vi "Extend Symbol Path_lvcicd.vi"(3 "Symbol Path":path) -> (1 "Resolved Path":path)   [LabVIEW 2014, in "_lvcicd_support_2014.lvlib"]
doc: "NEVSTOP-Programming-Palette 2022.3.9.1\nNEVSTOP - NEVSTOP\nCopyright (c) 2022, NEVSTOP"
uses:
  <vilib>/Utility/sysdir.llb/System Directory Type.ctl
  <userlib>/_OpenG.lib/file/file.llb/Valid Path - Traditional__ogtk.vi
  _lvcicd_support_2014.lvlib
  kernel32.dll
panel:
  # "#Note [xxx] or <xxx>\n- [application]\n- [desktop]\n- [temp][temporary]\n- [user.lib]\n- [vi.lib]\n-%SystemVariable%, eg: OneDrive"
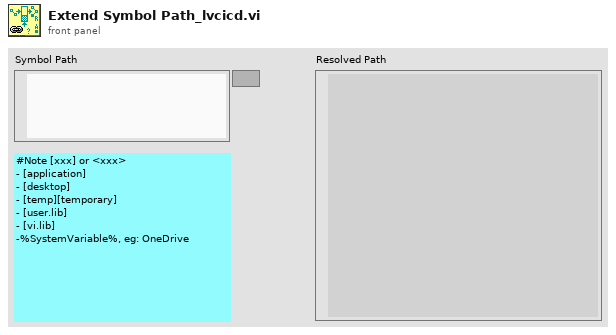
[diagram p1: front panel]
types:
  T1 = enum16{"Absolute path", "Relative path", "<Not A Path>"}
  T2 = typedef "System Directory Type.ctl" = i32
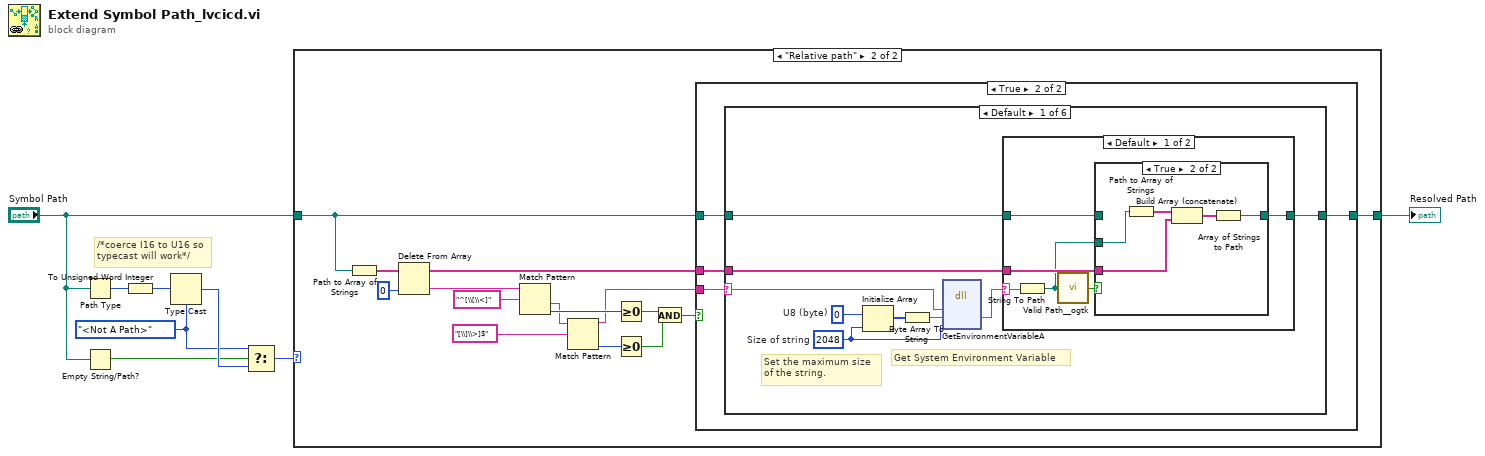
[diagram p0: block diagram]
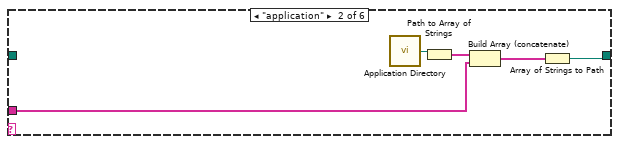
[diagram p6: hidden frame]
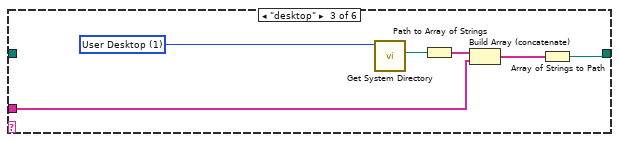
[diagram p7: hidden frame]
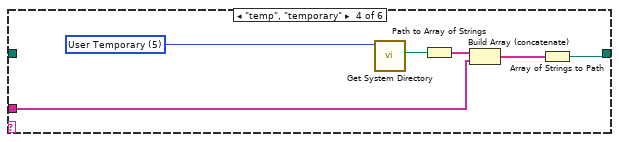
[diagram p8: hidden frame]
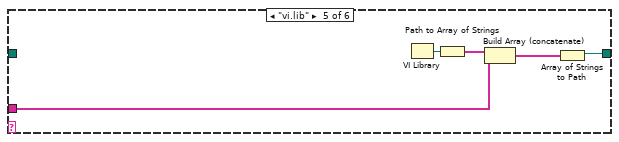
[diagram p9: hidden frame]
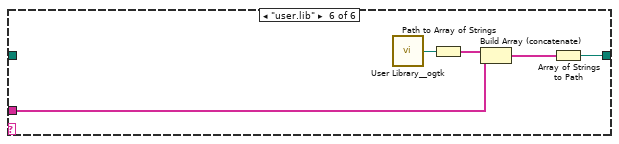
[diagram p10: hidden frame]
diagram:
  w3 = T1."<Not A Path>"
  # "/*coerce I16 to U16 so typecast will work*/"
  n1 = Path Type(1:"Symbol Path") -> (0:w1:i16)
  n2 = Empty String/Path?(string/path="Symbol Path") -> (empty?=w2:bool)
  n3 = To Unsigned Word Integer(number=w1) -> (unsigned 16bit integer=w5:u16)
  n4 = Type Cast(type=w3, x=w5) -> (*(type *) &x=w4:T1)
  n5 = Select(t=w3, s=w2, f=w4) -> (s? t:f=w8:T1)
  n6 = case shown="\"Relative path\"" w8 {
    tunnel: [w9 w16] -> w7
    tunnel: "Symbol Path" -> [w9 w15]
    frame "Absolute path", "<Not A Path>", Default {
    }
    frame "Relative path" {
      n7 = Path to Array of Strings(0:w15) -> (2:w24:string[])  [unwired: 1 out]
      n8 = Delete From Array(array=w24, index=0) -> (deleted portion=w14:string, array with subset deleted=w10:string[])  [unwired: 1 in]
      n9 = Match Pattern(string=w14, regular expression="^[\\[\\<]") -> (after substring=w13:string, offset past match=w21:i32)  [unwired: 1 in, 2 out]
      n10 = Match Pattern(string=w13, regular expression="[\\]\\>]$") -> (before substring=w12:string, offset past match=w20:i32)  [unwired: 1 in, 2 out]
      n11 = Greater Or Equal To 0?(x=w21) -> (x >= 0?=w19:bool)
      n12 = Greater Or Equal To 0?(x=w20) -> (x >= 0?=w18:bool)
      n13 = And(x=w19, y=w18) -> (x .and. y?=w17:bool)
      n14 = case shown="True" w17 {
        tunnel: [w25 w26] -> w16
        tunnel: w15 -> [w25 w28]
        tunnel: w12 -> [_ w29]
        tunnel: w10 -> [_ w27]
        frame False {
        }
        frame True {
          n15 = case shown="Default" w29 {
            selector: w29 -> [w38 _ _ _ _ _]
            tunnel: w28 -> [w35 _ _ _ _ _]
            tunnel: w27 -> [w34 w52 w59 w65 w69 w74]
            tunnel: [w36 w54 w60 w66 w71 w76] -> w26
            frame Default {
              w31 = u8 0  # U8 (byte)
              w30 = 2048  # Size of string
              # "Set the maximum size\nof the string."
              # "Get System Environment Variable"
              n16 = Initialize Array(w31, w30) -> (w32:u8[])
              n17 = Byte Array To String(unsigned byte array=w32) -> (string=w33:string)
              n18 = dll-call lib="kernel32.dll" fn="GetEnvironmentVariableA"("EnvVarName"=w38, "lpBuffer"=w33, "namelength"=w30) -> ("lpBuffer"=w37:string)  [unwired: 6 in, 2 out]
              n19 = case shown="Default" w37 {
                selector: w37 -> [w44 _]
                tunnel: [w42 w51] -> w36
                tunnel: w35 -> [w41 w51]
                tunnel: w34 -> [w40 _]
                frame Default {
                  n20 = String To Path(string=w44) -> (path=w39:path)
                  n21 = call-poly <userlib>:"Valid Path__ogtk.vi"("path"=w39) -> ("valid"=w43:bool)
                  n22 = case shown="True" w43 {
                    tunnel: [w45 w48] -> w42
                    tunnel: w41 -> [w45 _]
                    tunnel: w40 -> [_ w47]
                    tunnel: w39 -> [_ w46]
                    frame False {
                    }
                    frame True {
                      n23 = Path to Array of Strings(0:w46) -> (2:w49:string[])  [unwired: 1 out]
                      n24 = Build Array (concatenate)(w49, w47) -> (w50:string[])
                      n25 = Array of Strings to Path(0:w50) -> (2:w48:path)  [unwired: 1 in]
                    }
                  }
                }
                frame "" {
                }
              }
            }
            frame "application" {
              n26 = call <vilib>:"Application Directory.vi"() -> ("Application Directory"=w53:path)
              n27 = Path to Array of Strings(0:w53) -> (2:w55:string[])  [unwired: 1 out]
              n28 = Build Array (concatenate)(w55, w52) -> (w56:string[])
              n29 = Array of Strings to Path(0:w56) -> (2:w54:path)  [unwired: 1 in]
            }
            frame "desktop" {
              w58 = T2 1 items=["User Home"=0, "User Desktop"=1, "User Documents"=2, "User Application Data"=3, "User Preferences"=4, "User Temporary"=5, "Public Documents"=6, "Public Application Data"=7, "Public Preferences"=8, "Public Cache"=13, "System Core Libraries"=9, "System Installed Libraries"=10, "Application Files"=11, "Boot Volume Root"=12] ("system directory type")
              n30 = call <vilib>:"Get System Directory.vi"("system directory type"=w58) -> ("system directory"=w57:path)  [unwired: 10 in]
              n31 = Path to Array of Strings(0:w57) -> (2:w61:string[])  [unwired: 1 out]
              n32 = Build Array (concatenate)(w61, w59) -> (w62:string[])
              n33 = Array of Strings to Path(0:w62) -> (2:w60:path)  [unwired: 1 in]
            }
            frame "temp", "temporary" {
              w64 = T2 5 items=["User Home"=0, "User Desktop"=1, "User Documents"=2, "User Application Data"=3, "User Preferences"=4, "User Temporary"=5, "Public Documents"=6, "Public Application Data"=7, "Public Preferences"=8, "Public Cache"=13, "System Core Libraries"=9, "System Installed Libraries"=10, "Application Files"=11, "Boot Volume Root"=12] ("system directory type")
              n34 = call <vilib>:"Get System Directory.vi"("system directory type"=w64) -> ("system directory"=w63:path)  [unwired: 10 in]
              n35 = Path to Array of Strings(0:w63) -> (2:w67:string[])  [unwired: 1 out]
              n36 = Build Array (concatenate)(w67, w65) -> (w68:string[])
              n37 = Array of Strings to Path(0:w68) -> (2:w66:path)  [unwired: 1 in]
            }
            frame "vi.lib" {
              n38 = VI Library() -> (path=w70:path)
              n39 = Path to Array of Strings(0:w70) -> (2:w72:string[])  [unwired: 1 out]
              n40 = Build Array (concatenate)(w72, w69) -> (w73:string[])
              n41 = Array of Strings to Path(0:w73) -> (2:w71:path)  [unwired: 1 in]
            }
            frame "user.lib" {
              n42 = call <userlib>:"User Library__ogtk.vi"() -> ("User Library (+ Relative)"=w75:path)  [unwired: 1 in]
              n43 = Path to Array of Strings(0:w75) -> (2:w77:string[])  [unwired: 1 out]
              n44 = Build Array (concatenate)(w77, w74) -> (w78:string[])
              n45 = Array of Strings to Path(0:w78) -> (2:w76:path)  [unwired: 1 in]
            }
          }
        }
      }
    }
  }
  "Resolved Path" <- w7
